vi "forLAB.vi"() -> ()   [LabVIEW 2023]
uses:
  <vilib>/Analysis/NI_AALBase.lvlib
  <vilib>/Utility/file.llb/Write Delimited Spreadsheet (DBL).vi
panel:
  out "Waveform Chart":dbl(graph)
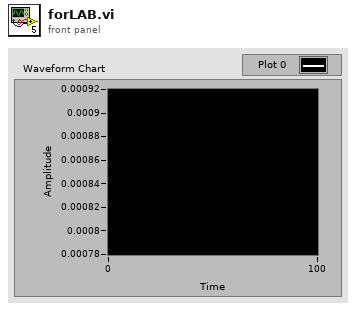
[diagram p1: front panel]
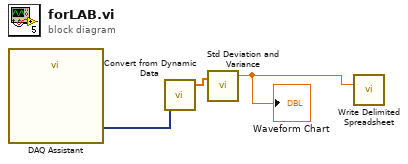
[diagram p0: block diagram]
diagram:
  n1 = call "DAQ Assistant"() -> ("data"=w3:dynamicdata)  [unwired: 17 in, 2 out]
  n2 = call "Convert from Dynamic Data"("Dynamic Data Type"=w3) -> ("Array"=w2:dbl[])  [unwired: 3 in]
  n3 = call <vilib>:"Std Deviation and Variance.vi"("X"=w2) -> ("mean"=w1:dbl)  [unwired: 1 in, 2 out]
  "Waveform Chart" <- w1
  n4 = call-poly <vilib>:"Write Delimited Spreadsheet.vi"("2D data"=w1) -> ()  [unwired: 13 in, 2 out]
